vi "Write.vi"(8 "error in (no error)":errorcluster, 9 "Variant":variant, 10 "String":string, 11 "RS232 in":refnum<class "RS-xxx.lvclass">) -> (0 "error out":errorcluster, 3 "RS232 out":refnum<class "RS-xxx.lvclass">)   [LabVIEW 2019, in "Protocols.lvlib" / "RS-xxx.lvclass"]
uses:
  RS-xxx.lvclass
  RS-xxx.lvclass/RS-xxx.ctl
  Data Access/Read Port Ref.vi
  Data Access/Write Port Ref.vi
  <vilib>/Utility/error.llb/Clear Errors.vi
  Protocols.lvlib
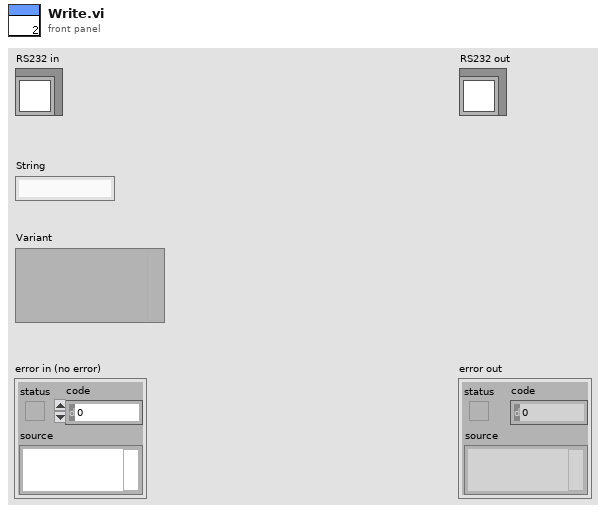
[diagram p1: front panel]
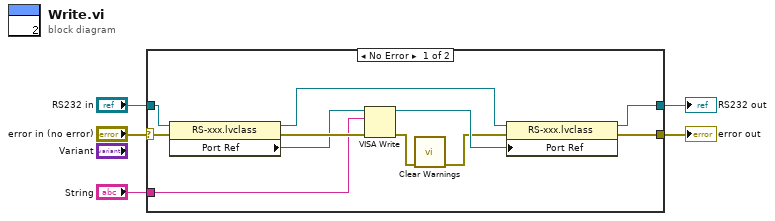
[diagram p0: block diagram]
diagram:
  n1 = case shown="No Error" "error in (no error)" {
    selector: "error in (no error)" -> [w8 w18]
    tunnel: "RS232 in" -> [w16 w17]
    tunnel: "String" -> [w14 _]
    tunnel: [w11 w18] -> w3
    tunnel: [w9 w17] -> w2
    frame No Error {
      n2 = property class="RS-xxx.lvclass"(reference=w16, error in=w8) -> (reference out=w10:refnum<class "RS-xxx.lvclass">, error out=w15:errorcluster, "Port Ref"=w13:refnum<visa-resource-name>)
      n3 = VISA Write(VISA resource name=w13, write buffer=w14, error in (no error)=w15) -> (VISA resource name out=w12:refnum<visa-resource-name>, error out=w7:errorcluster)  [unwired: 1 out]
      n4 = call "Clear Warnings.vi"("error in (no error)"=w7) -> ("error out"=w6:errorcluster)  [unwired: 10 in]
      n5 = property class="RS-xxx.lvclass"(reference=w10, error in=w6, "Port Ref"=w12) -> (reference out=w9:refnum<class "RS-xxx.lvclass">, error out=w11:errorcluster)
    }
    frame Error {
    }
  }
  "error out" <- w3
  "RS232 out" <- w2
